vi "Teleop.vi"(10 "Match Info":T1={"Autonomous Elapsed Seconds"=0.0, "TeleOp Elapsed Seconds"=0.0, "Disabled Elapsed Seconds"=0.0, "Visited Autonomous"=FALSE, "Visited TeleOp"=FALSE, "Visited Disabled"=FALSE, "Autonomous Settings"={"Autonomous Style"=enum."Independent", "VI Refnum"=refnum}}, 11 "Call Context":T2) -> ()   [LabVIEW 2020]
doc: "This VI is called for each enabled TeleOp packet received from the DS. It is typically used to read from joysticks and other inputs and update I/O or setpoints for timed control loops. It should complete and return within 20 milliseconds or risk missing DS packets."
uses:
  <vilib>/Rock Robotics/WPI/DriverStation/WPI_DriverStationDerivedRobotMode.ctl
  <vilib>/Rock Robotics/WPI/DriverStation/WPI_DriverStationMatch Info.ctl
  <vilib>/Rock Robotics/WPI/Utilities/WPI_GetSetVariantRefNum.vi
  <vilib>/Rock Robotics/Network Tables/NT Write Boolean Array.vi
  <vilib>/Rock Robotics/Network Tables/NT Write Numeric Array.vi
  Framework/Robot Global Data.vi
panel:
  out "TargetValid":bool
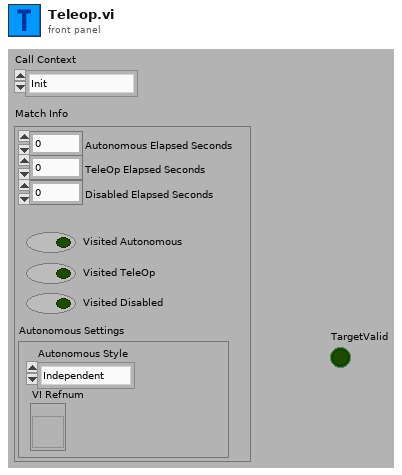
[diagram p1: front panel]
types:
  T1 = typedef "WPI_DriverStationMatch Info.ctl" = cluster{"Autonomous Elapsed Seconds":dbl, "TeleOp Elapsed Seconds":dbl, "Disabled Elapsed Seconds":dbl, "Visited Autonomous":bool, "Visited TeleOp":bool, "Visited Disabled":bool, "Autonomous Settings":cluster{"Autonomous Style":enum16{"Iterative", "Independent"}, "VI Refnum":refnum<vi>}}
  T2 = typedef "WPI_DriverStationDerivedRobotMode.ctl" = enum16{"Init", "Execute", "Stop"}
  T3 = typedef "WPI_JoystickDevRef.ctl" = cluster{"Device":T4}
  T4 = typedef "WPI_JoystickDeviceEnum.ctl" = enum16{"USB 0", "USB 1", "USB 2", "USB 3", "USB 4", "USB 5"}
  T5 = typedef "Command Status Info.ctl" = cluster{"Name":string, "Status":T6, "notifier out":T7}
  T6 = typedef "Completion Status.ctl" = enum16{"Successful", "Aborted", "Incomplete"}
  T7 = typedef "Completion Notifier.ctl" = refnum<notifier>
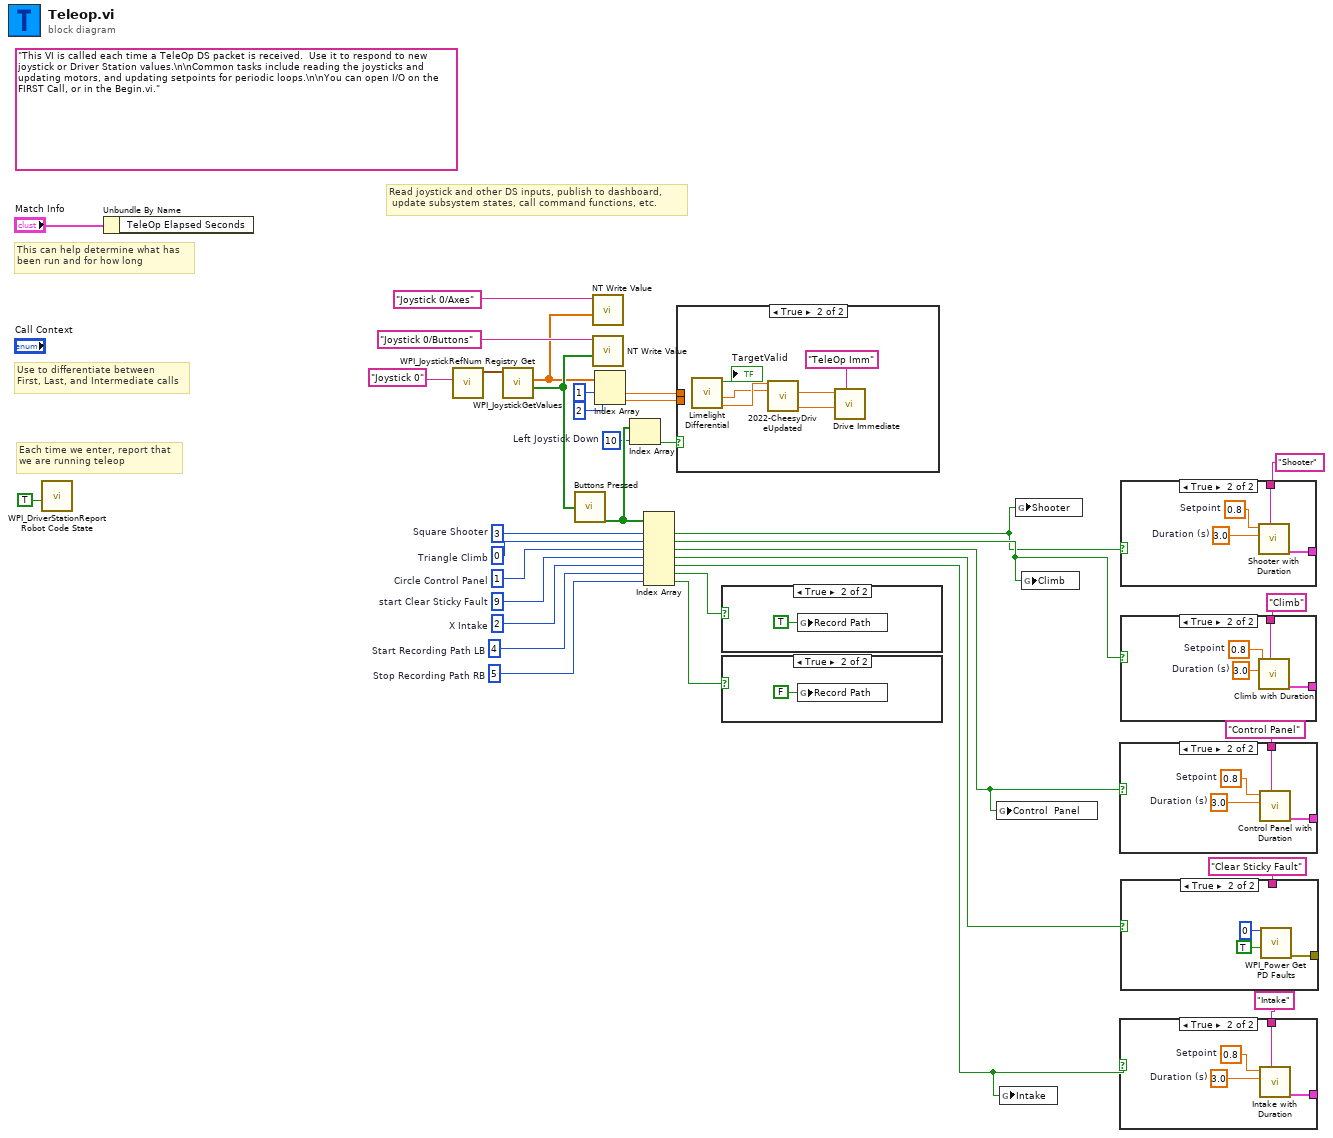
[diagram p0: block diagram]
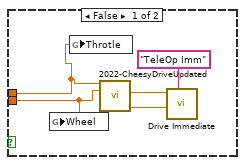
[diagram p2: hidden frame]
diagram:
  w1 = 10  # Left Joystick Down
  w6 = 5  # Stop Recording Path RB
  w7 = 4  # Start Recording Path LB
  w15 = 2  # X Intake
  w19 = 9  # start Clear Sticky Fault
  w22 = 1  # Circle Control Panel
  w23 = 0  # Triangle Climb
  w24 = 3  # Square Shooter
  (unwired) "This VI is called each time a TeleOp DS packet is received.  Use it to respond to new joystick or Driver Station values.\n\nCommon tasks include reading the joysticks and updating motors, and updating setpoints for periodic loops.\n\nYou can open I/O on the FIRST Call, or in the Begin.vi."
  # "Read joystick and other DS inputs, publish to dashboard,\n update subsystem states, call command functions, etc."
  # "Each time we enter, report that\nwe are running teleop"
  # "Use to differentiate between\nFirst, Last, and Intermediate calls"
  # "This can help determine what has\nbeen run and for how long"
  n1 = call <vilib>:"WPI_DriverStationReport Robot Code State.vi"("TeleOp"=TRUE ("Autonomous")) -> ()  [unwired: 10 in, 1 out]
  n2 = Unbundle By Name("Match Info") -> ()  [unwired: 1 out]
  n3 = call <vilib>:"WPI_JoystickRefNum Registry Get.vi"("refnum name"="Joystick 0") -> ("JoystickDevRef"=w31:T3)  [unwired: 1 in, 9 out]
  n4 = call <vilib>:"WPI_JoystickGetValues.vi"("JoystickDevRef"=w31) -> ("Buttons"=w27:bool[], "Axes"=w26:dbl[])  [unwired: 6 in, 3 out]
  n5 = call "Buttons Pressed.vi"("Button Values"=w27) -> ("Button Presses"=w3:bool[])
  n6 = call-poly <vilib>:"NT Write Value.vi"("Numeric Array"=w26, "Name"="Joystick 0/Axes") -> ()  [unwired: 9 in, 1 out]
  n7 = call-poly <vilib>:"NT Write Value.vi"("Boolean Array"=w27, "Name"="Joystick 0/Buttons") -> ()  [unwired: 9 in, 1 out]
  n8 = Index Array(array=w26, index #1=1 ("index"), index #2=2 ("index")) -> (element #1=w9:dbl, element #2=w8:dbl)
  n9 = Index Array(array=w3, index=w1) -> (element=w2:bool)
  n10 = Index Array(array=w3, index #1=w24, index #2=w23, index #3=w22, index #4=w19, index #5=w15, index #6=w7, index #7=w6) -> (element #1=w10:bool, element #2=w11:bool, element #3=w12:bool, element #4=w18:bool, element #5=w13:bool, element #6=w5:bool, element #7=w4:bool)
  n11 = case shown="True" w2 {
    tunnel: w9 -> [w36 _]
    tunnel: w8 -> [w35 _]
    frame False {
      n12 = global write "Robot Global Data.vi" "Wheel"(w35) -> ()
      n13 = global write "Robot Global Data.vi" "Throtle"(w36) -> ()
      n14 = call "2022-CheesyDriveUpdated.vi"("Throttle"=w36, "Wheel"=w35) -> ("Left PWM"=w38:dbl, "Right PWM"=w37:dbl)  [unwired: 11 in, 1 out]
      n15 = call "Drive Immediate.vi"("Description"="TeleOp Imm", "Right Setpoint"=w37, "Left Setpoint"=w38) -> ()  [unwired: 8 in, 1 out]
    }
    frame True {
      n16 = call "Limelight Differential.vi"() -> ("DriveCommand"=w42:dbl, "SteerCommand"=w41:dbl, "TargetValid"=→"TargetValid":bool)  [unwired: 9 in]
      n17 = call "2022-CheesyDriveUpdated.vi"("Throttle"=w42, "Wheel"=w41) -> ("Left PWM"=w44:dbl, "Right PWM"=w43:dbl)  [unwired: 11 in, 1 out]
      n18 = call "Drive Immediate.vi"("Description"="TeleOp Imm", "Right Setpoint"=w43, "Left Setpoint"=w44) -> ()  [unwired: 8 in, 1 out]
    }
  }
  n19 = case shown="True" w5 {
    frame False {
    }
    frame True {
      n20 = global write "Robot Global Data.vi" "Record Path"(TRUE ("Record Path")) -> ()
    }
  }
  n21 = case shown="True" w4 {
    frame False {
    }
    frame True {
      n22 = global write "Robot Global Data.vi" "Record Path"(FALSE ("Record Path")) -> ()
    }
  }
  n23 = global write "Robot Global Data.vi" "Control  Panel"(w12) -> ()
  n24 = global write "Robot Global Data.vi" "Intake"(w13) -> ()
  n25 = global write "Robot Global Data.vi" "Shooter"(w10) -> ()
  n26 = global write "Robot Global Data.vi" "Climb"(w11) -> ()
  n27 = case shown="True" w12 {
    tunnel: [_ w51] -> _
    tunnel: "Control Panel" ("Description") -> [_ w50]
    frame False {
    }
    frame True {
      w48 = 3.0  # Duration (s)
      w49 = 0.8  # Setpoint
      n28 = call "Control Panel with Duration.vi"("Description"=w50, "Duration (s)"=w48, "Setpoint"=w49) -> ("Command Info Out"=w51:T5)  [unwired: 8 in]
    }
  }
  n29 = case shown="True" w13 {
    tunnel: [_ w55] -> _
    tunnel: "Intake" ("Description") -> [_ w54]
    frame False {
    }
    frame True {
      w52 = 3.0  # Duration (s)
      w53 = 0.8  # Setpoint
      n30 = call "Intake with Duration.vi"("Description"=w54, "Duration (s)"=w52, "Setpoint"=w53) -> ("Command Info Out"=w55:T5)  [unwired: 8 in]
    }
  }
  n31 = case shown="True" w10 {
    tunnel: [_ w59] -> _
    tunnel: "Shooter" ("Description") -> [_ w58]
    frame False {
    }
    frame True {
      w56 = 3.0  # Duration (s)
      w57 = 0.8  # Setpoint
      n32 = call "Shooter with Duration.vi"("Description"=w58, "Duration (s)"=w56, "Setpoint"=w57) -> ("Command Info Out"=w59:T5)  [unwired: 8 in]
    }
  }
  n33 = case shown="True" w11 {
    tunnel: [_ w63] -> _
    tunnel: "Climb" ("Description") -> [_ w62]
    frame False {
    }
    frame True {
      w60 = 0.8  # Setpoint
      w61 = 3.0  # Duration (s)
      n34 = call "Climb with Duration.vi"("Description"=w62, "Duration (s)"=w61, "Setpoint"=w60) -> ("Command Info Out"=w63:T5)  [unwired: 8 in]
    }
  }
  n35 = case shown="True" w18 {
    tunnel: [_ w66] -> _
    tunnel: "Clear Sticky Fault" ("Description") -> [_ _]
    frame False {
    }
    frame True {
      n36 = call <vilib>:"WPI_Power Get PD Faults.vi"("Power Distribution (def)"=u8 0, "Clear Sticky Faults"=TRUE) -> ("error out"=w66:errorcluster)  [unwired: 10 in, 3 out]
    }
  }
